vi "子VI-检测模式配置.vi"() -> (0 "视频检测帧间隔output":i8, 1 "模式选择output":i8, 2 "是否使用GPU计算output":i8, 3 "图片/视频路径":string, 4 "flag":i32, 5 "图片/视频完整路径":path)   [LabVIEW 2018]
panel:
  in  "确认":bool
  in  "视频检测帧间隔":i8
  in  "是否使用GPU计算":i8(ring) items=["否", "是"]
  in  "模式选择":i8(ring) items=["单张图片检测", "视频检测"]
  # "检测信息配置"
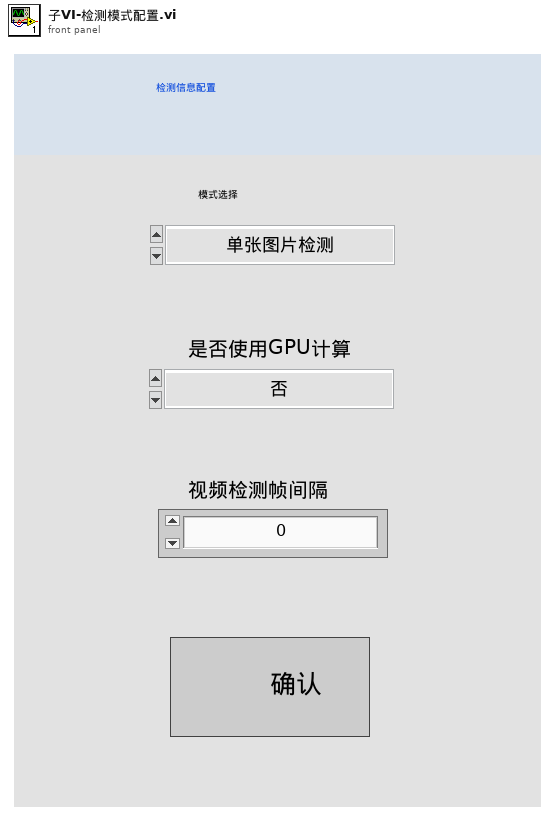
[diagram p1: front panel]
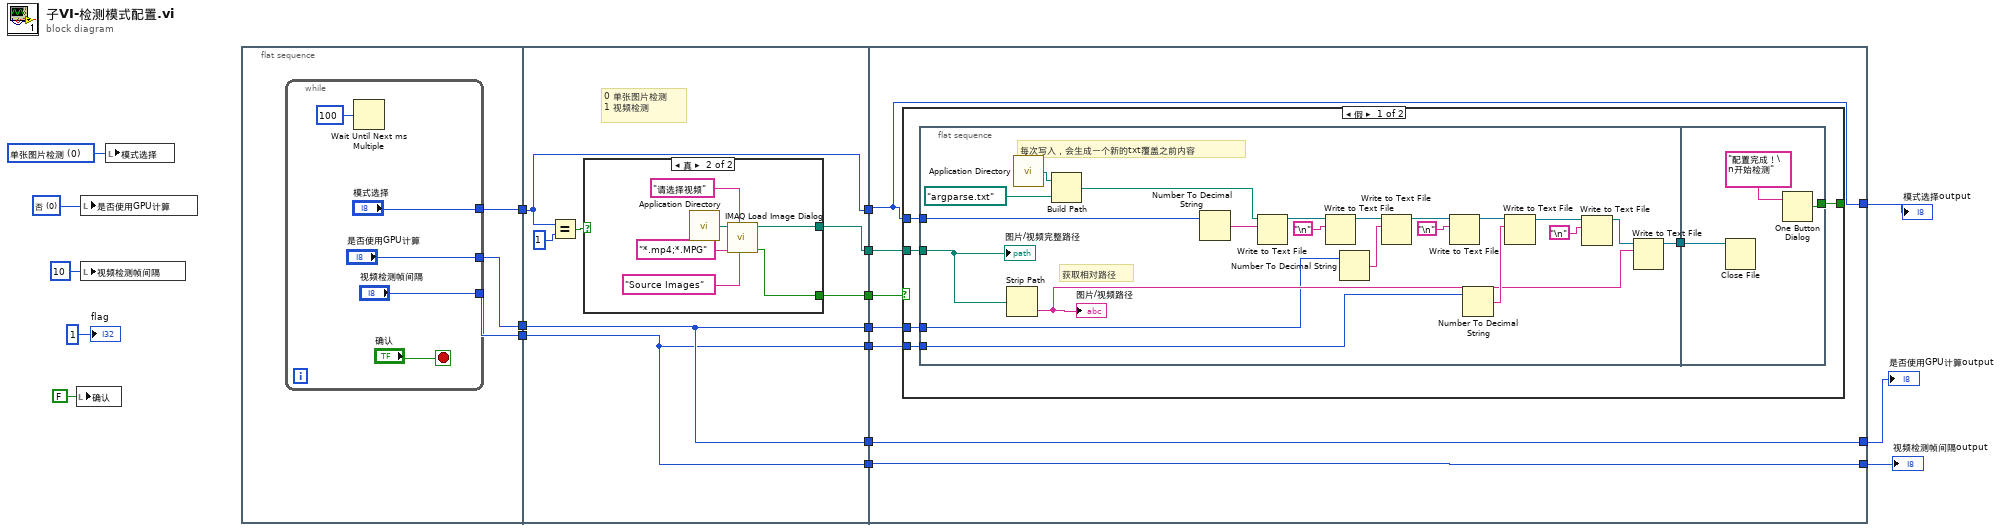
[diagram p0: block diagram]
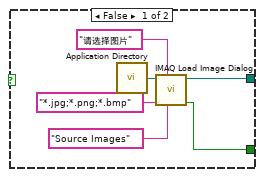
[diagram p2: hidden frame]
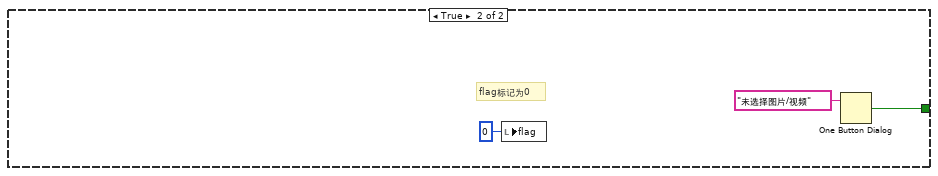
[diagram p3: hidden frame]
diagram:
  w17 = u16 0 items=["否", "是"] ("是否使用GPU计算")
  w18 = u16 0 items=["单张图片检测", "视频检测"] ("模式选择")
  n1 = local write "确认"(FALSE ("确认")) -> ()
  n2 = local write "是否使用GPU计算"(w17) -> ()
  n3 = local write "视频检测帧间隔"(u16 10 ("视频检测帧间隔")) -> ()
  n4 = local write "模式选择"(w18) -> ()
  n5 = flat-sequence {
    tunnel: [w21] -> w15
    tunnel: [w20] -> w14
    tunnel: [w19] -> w13
    tunnel: w15 -> [w32]
    tunnel: [w32] -> w12
    tunnel: w14 -> [w28]
    tunnel: [w28] -> w11
    tunnel: w13 -> [w27]
    tunnel: [w27] -> w10
    tunnel: [w30] -> w9
    tunnel: [w29] -> w8
    tunnel: [w28] -> w7
    tunnel: [w27] -> w6
    tunnel: w12 -> [w46]
    tunnel: w11 -> [w52]
    tunnel: w10 -> [w51]
    tunnel: w9 -> [w49]
    tunnel: w8 -> [w50]
    tunnel: [w52] -> w4
    tunnel: [w51] -> w3
    tunnel: [w46] -> w5
    tunnel: w7 -> [w48]
    tunnel: w6 -> [w47]
    frame #0 {
      n6 = while {
        tunnel: ["模式选择"] -> w21
        tunnel: ["是否使用GPU计算"] -> w20
        tunnel: ["视频检测帧间隔"] -> w19
        stop <- "确认" stop-if-true
        n7 = Wait Until Next ms Multiple(millisecond multiple=u32 100 ("毫秒倍数")) -> ()  [unwired: 1 out]
      }
    }
    frame #1 {
      # "0 单张图片检测\n1 视频检测"
      n8 = Equal?(x=w32, y=i8 1) -> (x = y?=w31:bool)
      n9 = case shown="真" w31 {
        tunnel: [w35 w41] -> w30
        tunnel: [w34 w40] -> w29
        frame False {
          n10 = call <vilib>:"Application Directory.vi"() -> ("Application Directory"=w39:path)
          n11 = call "IMAQ Load Image Dialog"("Pattern Label"="Source Images", "Prompt"="请选择图片" ("prompt"), "Pattern"="*.jpg;*.png;*.bmp", "Start Path"=w39) -> ("Cancelled?"=w34:bool, "Path"=w35:path)  [unwired: 5 in, 1 out]
        }
        frame True {
          n12 = call <vilib>:"Application Directory.vi"() -> ("Application Directory"=w45:path)
          n13 = call "IMAQ Load Image Dialog"("Pattern Label"="Source Images", "Prompt"="请选择视频" ("prompt"), "Pattern"="*.mp4;*.MPG", "Start Path"=w45) -> ("Cancelled?"=w40:bool, "Path"=w41:path)  [unwired: 5 in, 1 out]
        }
      }
    }
    frame #2 {
      n14 = case shown="假" w50 {
        tunnel: w49 -> [w58 _]
        tunnel: [w53 w85] -> _
        tunnel: w48 -> [w56 _]
        tunnel: w47 -> [w55 _]
        tunnel: w46 -> [w54 _]
        frame False {
          n15 = flat-sequence {
            tunnel: w58 -> [w63]
            tunnel: [w62] -> w57
            tunnel: w56 -> [w61]
            tunnel: w55 -> [w60]
            tunnel: w54 -> [w59]
            tunnel: w57 -> [w81]
            tunnel: [w80] -> w53
            frame #0 {
              # "获取相对路径"
              # "每次写入，会生成一个新的txt覆盖之前内容"
              n16 = Strip Path(path=w63) -> (name=w64:string)  [unwired: 1 out]
              "图片/视频路径" <- w64
              n17 = call <vilib>:"Application Directory.vi"() -> ("Application Directory"=w76:path)
              n18 = Build Path(base path=w76, name or relative path=path "argparse.txt" ("文件（使用对话框）")) -> (appended path=w68:path)
              n19 = Number To Decimal String(number=w59) -> (decimal integer string=w79:string)  [unwired: 1 in]
              n20 = Write to Text File(file (use dialog)=w68, text=w79) -> (refnum out=w72:refnum<file>)  [unwired: 2 in, 2 out]
              n21 = Write to Text File(file (use dialog)=w72, text="\n") -> (refnum out=w71:refnum<file>)  [unwired: 2 in, 2 out]
              n22 = Number To Decimal String(number=w61) -> (decimal integer string=w78:string)  [unwired: 1 in]
              n23 = Write to Text File(file (use dialog)=w71, text=w78) -> (refnum out=w70:refnum<file>)  [unwired: 2 in, 2 out]
              n24 = Write to Text File(file (use dialog)=w70, text="\n") -> (refnum out=w69:refnum<file>)  [unwired: 2 in, 2 out]
              n25 = Number To Decimal String(number=w60) -> (decimal integer string=w77:string)  [unwired: 1 in]
              n26 = Write to Text File(file (use dialog)=w69, text=w77) -> (refnum out=w66:refnum<file>)  [unwired: 2 in, 2 out]
              n27 = Write to Text File(file (use dialog)=w66, text="\n") -> (refnum out=w65:refnum<file>)  [unwired: 2 in, 2 out]
              n28 = Write to Text File(file (use dialog)=w65, text=w64) -> (refnum out=w62:refnum<file>)  [unwired: 2 in, 2 out]
              "图片/视频完整路径" <- w63
            }
            frame #1 {
              n29 = Close File(refnum=w81) -> ()  [unwired: 1 in, 2 out]
              n30 = One Button Dialog(message="配置完成！\n开始检测" ("消息")) -> (true=w80:bool)  [unwired: 1 in]
            }
          }
        }
        frame True {
          # "flag标记为0"
          n31 = local write "flag"(0 ("flag")) -> ()
          n32 = One Button Dialog(message="未选择图片/视频" ("消息")) -> (true=w85:bool)  [unwired: 1 in]
        }
      }
    }
  }
  "模式选择output" <- w5
  "是否使用GPU计算output" <- w4
  "视频检测帧间隔output" <- w3
  "flag" <- 1
